vi "Packet decoder - Telemetry.vi"(8 "error in (no error)":errorcluster, 9 "Data format":enum16{"IDRA data", "XAM data"}(ring), 10 "Packet array":u8[](array[numeric]), 11 "Input packet":T1) -> (0 "error out":errorcluster, 2 "Valid packet":bool, 3 "Output packet":T1)   [LabVIEW 2015, in "Acquisition.lvlib"]
uses:
  Acquisition.lvlib
  Generic data packet.ctl
  My Graphs/Gps Map Graph coordinates.ctl
  IDRA Data Packet.ctl
  XAM Data Packet.ctl
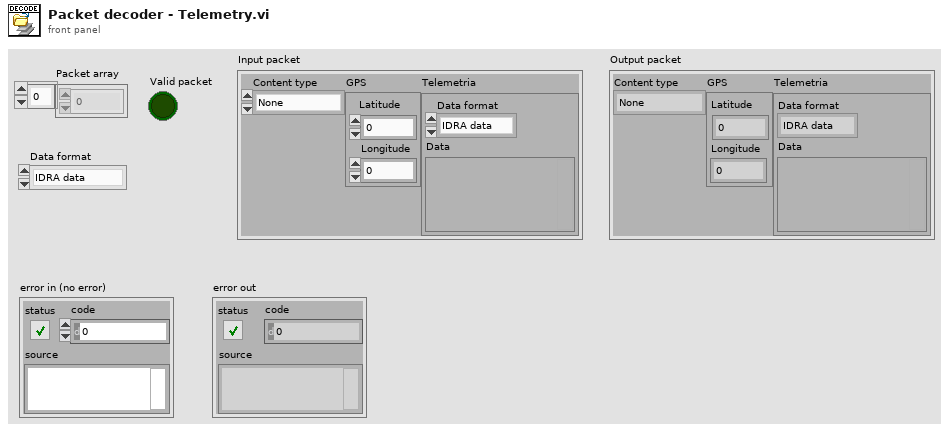
[diagram p1: front panel]
types:
  T1 = typedef "Acquisition.lvlib/Generic data packet.ctl" = cluster{"Content type":enum16{"None", "Telemetria", "GPS"}, "GPS":T2, "Telemetria":cluster{"Data format":enum16{"IDRA data", "XAM data"}, "Data":variant}}
  T2 = typedef "Gps Map Graph coordinates.ctl" = cluster{"Latitude":dbl, "Longitude":dbl}
  T3 = typedef "Acquisition.lvlib/IDRA Data Packet.ctl" = cluster{"Minutes":u16, "Seconds/100":u16, "Voltage":sgl, "Current":sgl, "Speed":sgl, "Temperature 1":sgl, "Temperature 2":sgl, "Temperature 3":sgl, "Humidity 1":sgl, "Humidity 2":sgl, "Strategy":u8, "Electric Motor":bool, "Electronics":bool, "Emergency":bool}
  T4 = typedef "Acquisition.lvlib/XAM Data Packet.ctl" = cluster{"Minutes":u16, "Seconds/100":u16, "Supercap Voltage":sgl, "Battery Voltage":sgl, "Supercap Current":sgl, "Speed":sgl, "EM Temperature":sgl, "ECU Temperature":sgl, "ICE Temperature":sgl, "RPM EM":u16, "RPM ICE":u16, "Cruise Control":bool, "Emergency":bool}
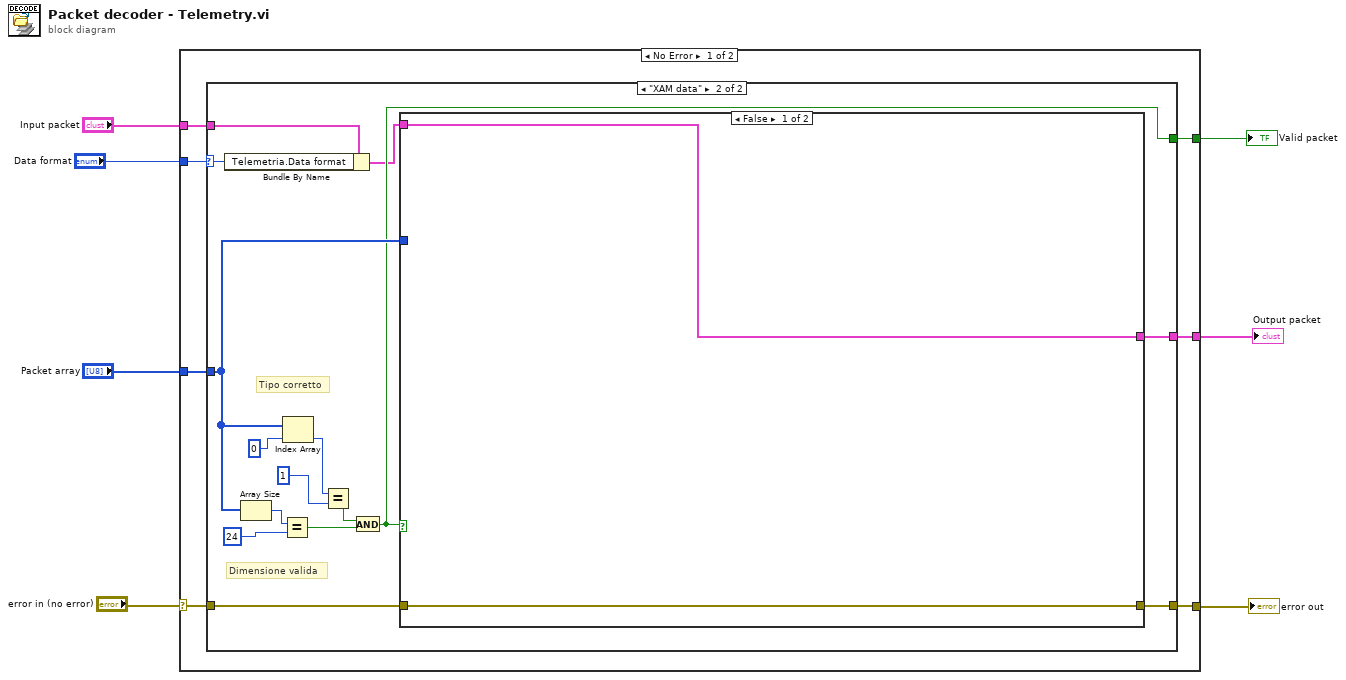
[diagram p0: block diagram]
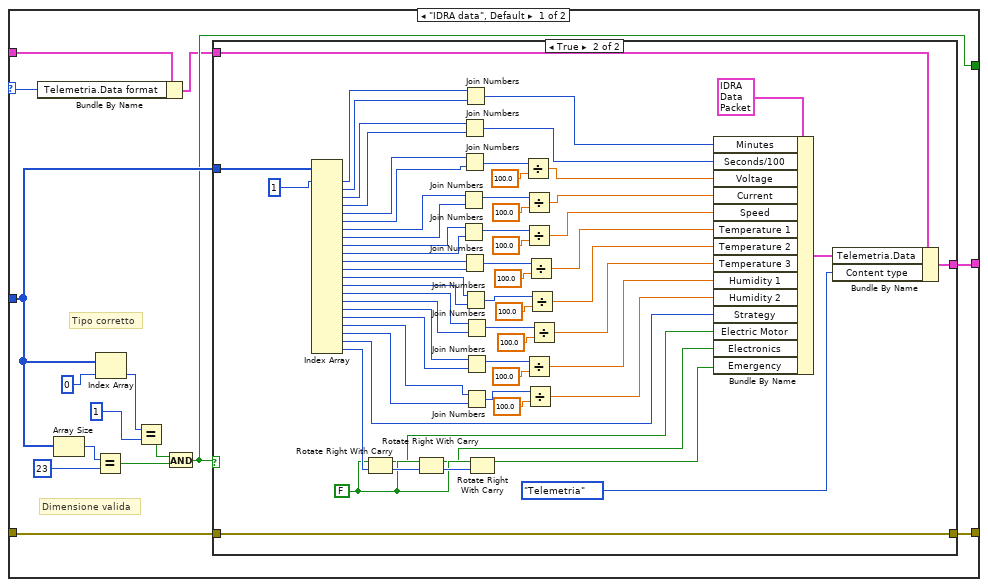
[diagram p2: hidden frame]
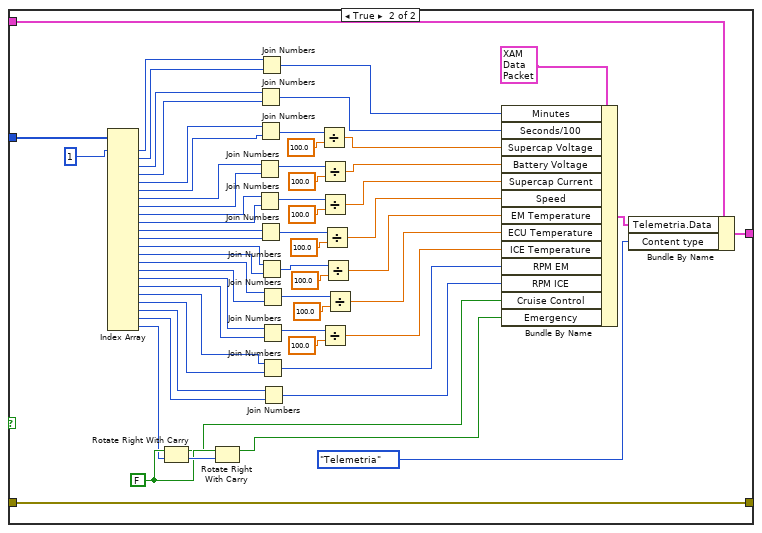
[diagram p4: hidden frame]
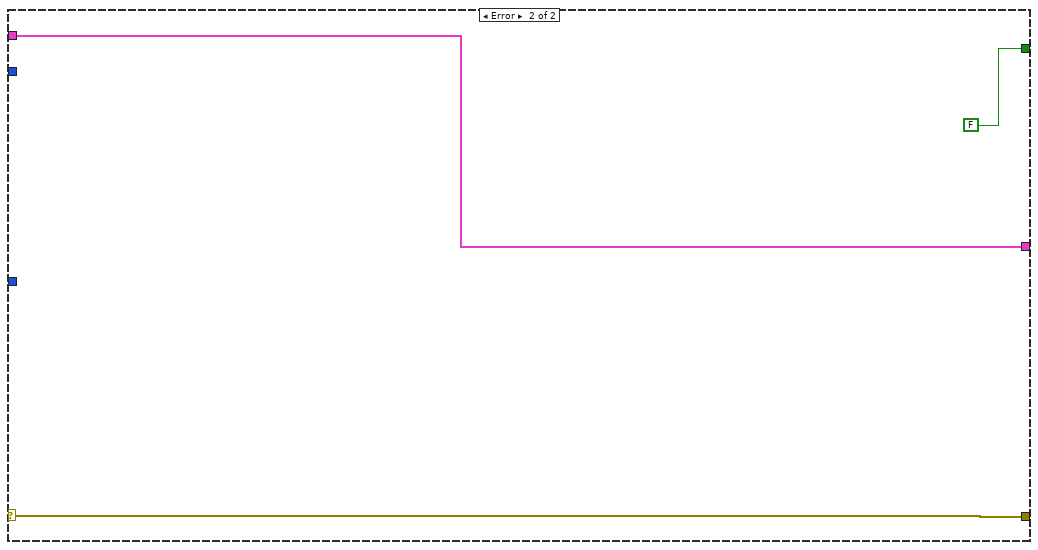
[diagram p5: hidden frame]
diagram:
  n1 = case shown="No Error" "error in (no error)" {
    selector: "error in (no error)" -> [w12 w171]
    tunnel: [w14 w172] -> w2
    tunnel: "Input packet" -> [w13 w172]
    tunnel: "Packet array" -> [w10 _]
    tunnel: [w11 w171] -> w5
    tunnel: [w9 FALSE] -> w4
    tunnel: "Data format" -> [w8 _]
    frame No Error {
      n2 = case shown="\"XAM data\"" w8 {
        selector: w8 -> [w17 w97]
        tunnel: [w20 w108] -> w14
        tunnel: w13 -> [w18 w96]
        tunnel: w12 -> [w22 w106]
        tunnel: [w21 w105] -> w11
        tunnel: w10 -> [w23 w104]
        tunnel: [w19 w98] -> w9
        frame "IDRA data", Default {
          # "Tipo corretto"
          # "Dimensione valida"
          n3 = Bundle By Name(cluster=w18, "Telemetria.Data format"=w17) -> (w16:T1)
          n4 = Array Size(array=w23) -> (size(s)=w29:i32)
          n5 = Equal?(x=w29, y=23) -> (x = y?=w27:bool)
          n6 = Index Array(array=w23, index=0) -> (element=w25:u8)
          n7 = Equal?(x=w25, y=u8 1) -> (x = y?=w26:bool)
          n8 = And(x=w26, y=w27) -> (x .and. y?=w19:bool)
          n9 = case shown="True" w19 {
            tunnel: [w31 w34] -> w20
            tunnel: w16 -> [w31 w35]
            tunnel: w23 -> [_ w92]
            tunnel: w22 -> [w30 w91]
            tunnel: [w30 w91] -> w21
            frame False {
            }
            frame True {
              w40 = FALSE ("carry")
              n10 = Index Array(array=w92, index #1=1 ("index")) -> (element #1=w72:u8, element #2=w73:u8, element #3=w70:u8, element #4=w69:u8, element #5=w59:u8, element #6=w58:u8, element #7=w57:u8, element #8=w56:u8, element #9=w55:u8, element #10=w54:u8, element #11=w53:u8, element #12=w52:u8, element #13=w51:u8, element #14=w50:u8, element #15=w49:u8, element #16=w48:u8, element #17=w47:u8, element #18=w46:u8, element #19=w45:u8, element #20=w44:u8, element #21=w74:u8, element #22=w43:u8)  [unwired: 21 in]
              n11 = Rotate Right With Carry(2:w43, 3:w40) -> (0:w41:u8, 1:w39:bool)
              n12 = Rotate Right With Carry(2:w41, 3:w40) -> (0:w42:u8, 1:w38:bool)
              n13 = Join Numbers(hi=w57, lo=w56) -> ((hi.lo)=w66:u16)
              n14 = Join Numbers(hi=w55, lo=w54) -> ((hi.lo)=w65:u16)
              n15 = Join Numbers(hi=w70, lo=w69) -> ((hi.lo)=w68:u16)
              n16 = Join Numbers(hi=w59, lo=w58) -> ((hi.lo)=w67:u16)
              n17 = Join Numbers(hi=w53, lo=w52) -> ((hi.lo)=w64:u16)
              n18 = Join Numbers(hi=w72, lo=w73) -> ((hi.lo)=w71:u16)
              n19 = Join Numbers(hi=w51, lo=w50) -> ((hi.lo)=w63:u16)
              n20 = Join Numbers(hi=w49, lo=w48) -> ((hi.lo)=w62:u16)
              n21 = Join Numbers(hi=w47, lo=w46) -> ((hi.lo)=w61:u16)
              n22 = Join Numbers(hi=w45, lo=w44) -> ((hi.lo)=w60:u16)
              n23 = Rotate Right With Carry(2:w42, 3:w40) -> (1:w37:bool)  [unwired: 1 out]
              n24 = Divide(x=w67, y=100.0) -> (x/y=w89:dbl)
              n25 = Divide(x=w66, y=100.0) -> (x/y=w87:dbl)
              n26 = Divide(x=w65, y=100.0) -> (x/y=w85:dbl)
              n27 = Divide(x=w61, y=100.0) -> (x/y=w76:dbl)
              n28 = Divide(x=w60, y=100.0) -> (x/y=w75:dbl)
              n29 = Divide(x=w64, y=100.0) -> (x/y=w79:dbl)
              n30 = Divide(x=w63, y=100.0) -> (x/y=w78:dbl)
              n31 = Divide(x=w62, y=100.0) -> (x/y=w77:dbl)
              n32 = Bundle By Name "Bundle By Name"(cluster=T3 {"Minutes"=0, "Seconds/100"=0, "Voltage"=0.0, "Current"=0.0, "Speed"=0.0, "Temperature 1"=0.0, "Temperature 2"=0.0, "Temperature 3"=0.0, "Humidity 1"=0.0, "Humidity 2"=0.0, "Strategy"=0, "Electric Motor"=FALSE, "Electronics"=FALSE, "Emergency"=FALSE} ("IDRA Data Packet"), "Minutes"=w71, "Seconds/100"=w68, "Voltage"=w89, "Current"=w87, "Speed"=w85, "Temperature 1"=w79, "Temperature 2"=w78, "Temperature 3"=w77, "Humidity 1"=w76, "Humidity 2"=w75, "Strategy"=w74, "Electric Motor"=w39, "Electronics"=w38, "Emergency"=w37) -> (w33:T3)
              n33 = Bundle By Name(cluster=w35, "Telemetria.Data"=w33, "Content type"=enum16{"None", "Telemetria", "GPS"}."Telemetria" ("Enum")) -> (w34:T1)
            }
          }
        }
        frame "XAM data" {
          # "Tipo corretto"
          # "Dimensione valida"
          n34 = Bundle By Name(cluster=w96, "Telemetria.Data format"=w97) -> (w95:T1)
          n35 = Array Size(array=w104) -> (size(s)=w107:i32)
          n36 = Equal?(x=w107, y=24) -> (x = y?=w102:bool)
          n37 = Index Array(array=w104, index=0) -> (element=w100:u8)
          n38 = Equal?(x=w100, y=u8 1) -> (x = y?=w101:bool)
          n39 = And(x=w101, y=w102) -> (x .and. y?=w98:bool)
          n40 = case shown="False" w98 {
            tunnel: [w110 w119] -> w108
            tunnel: w95 -> [w110 w120]
            tunnel: w104 -> [_ w169]
            tunnel: w106 -> [w109 w168]
            tunnel: [w109 w168] -> w105
            frame False {
            }
            frame True {
              w123 = FALSE ("carry")
              n41 = Index Array(array=w169, index #1=1 ("index")) -> (element #1=w152:u8, element #2=w153:u8, element #3=w150:u8, element #4=w149:u8, element #5=w140:u8, element #6=w139:u8, element #7=w138:u8, element #8=w137:u8, element #9=w136:u8, element #10=w135:u8, element #11=w134:u8, element #12=w133:u8, element #13=w132:u8, element #14=w131:u8, element #15=w130:u8, element #16=w129:u8, element #17=w128:u8, element #18=w127:u8, element #19=w126:u8, element #20=w125:u8, element #21=w112:u8, element #22=w113:u8, element #23=w114:u8)  [unwired: 22 in]
              n42 = Rotate Right With Carry(2:w114, 3:w123) -> (0:w124:u8, 1:w122:bool)
              n43 = Rotate Right With Carry(2:w124, 3:w123) -> (1:w121:bool)  [unwired: 1 out]
              n44 = Join Numbers(hi=w138, lo=w137) -> ((hi.lo)=w146:u16)
              n45 = Join Numbers(hi=w136, lo=w135) -> ((hi.lo)=w145:u16)
              n46 = Join Numbers(hi=w150, lo=w149) -> ((hi.lo)=w148:u16)
              n47 = Join Numbers(hi=w140, lo=w139) -> ((hi.lo)=w147:u16)
              n48 = Join Numbers(hi=w134, lo=w133) -> ((hi.lo)=w144:u16)
              n49 = Join Numbers(hi=w152, lo=w153) -> ((hi.lo)=w151:u16)
              n50 = Join Numbers(hi=w132, lo=w131) -> ((hi.lo)=w143:u16)
              n51 = Join Numbers(hi=w130, lo=w129) -> ((hi.lo)=w142:u16)
              n52 = Join Numbers(hi=w128, lo=w127) -> ((hi.lo)=w141:u16)
              n53 = Join Numbers(hi=w126, lo=w125) -> ((hi.lo)=w115:u16)
              n54 = Join Numbers(hi=w112, lo=w113) -> ((hi.lo)=w111:u16)
              n55 = Divide(x=w147, y=100.0) -> (x/y=w166:dbl)
              n56 = Divide(x=w146, y=100.0) -> (x/y=w164:dbl)
              n57 = Divide(x=w145, y=100.0) -> (x/y=w162:dbl)
              n58 = Divide(x=w141, y=100.0) -> (x/y=w154:dbl)
              n59 = Divide(x=w144, y=100.0) -> (x/y=w157:dbl)
              n60 = Divide(x=w143, y=100.0) -> (x/y=w156:dbl)
              n61 = Divide(x=w142, y=100.0) -> (x/y=w155:dbl)
              n62 = Bundle By Name "Bundle By Name"(cluster=T4 {"Minutes"=0, "Seconds/100"=0, "Supercap Voltage"=0.0, "Battery Voltage"=0.0, "Supercap Current"=0.0, "Speed"=0.0, "EM Temperature"=0.0, "ECU Temperature"=0.0, "ICE Temperature"=0.0, "RPM EM"=0, "RPM ICE"=0, "Cruise Control"=FALSE, "Emergency"=FALSE} ("XAM Data Packet"), "Minutes"=w151, "Seconds/100"=w148, "Supercap Voltage"=w166, "Battery Voltage"=w164, "Supercap Current"=w162, "Speed"=w157, "EM Temperature"=w156, "ECU Temperature"=w155, "ICE Temperature"=w154, "RPM EM"=w115, "RPM ICE"=w111, "Cruise Control"=w122, "Emergency"=w121) -> (w118:T4)
              n63 = Bundle By Name(cluster=w120, "Telemetria.Data"=w118, "Content type"=enum16{"None", "Telemetria", "GPS"}."Telemetria" ("Enum")) -> (w119:T1)
            }
          }
        }
      }
    }
    frame Error {
    }
  }
  "error out" <- w5
  "Valid packet" <- w4
  "Output packet" <- w2
